vi "MAIN_launch_movie_acquisition.vi"(3 "error in":errorcluster, 4 "Data cluster":T3 {"Global parameters"."# repetitions" min=0; "Global parameters"."Dt (s)" min=0 step=1; "Global parameters"."Filter list" items=["ET665lp", "zet405/488/561/640m", "None", "None", "None", "None"]}, 5 "queue CAMERA":refnum<queue>) -> (1 "error out":errorcluster, 2 "Next task":T1)   [LabVIEW 2015]
uses:
  CONTROLS/Global parameters.ctl
  CONTROLS/Q_camera_element.ctl
  CONTROLS/Q_main_element.ctl
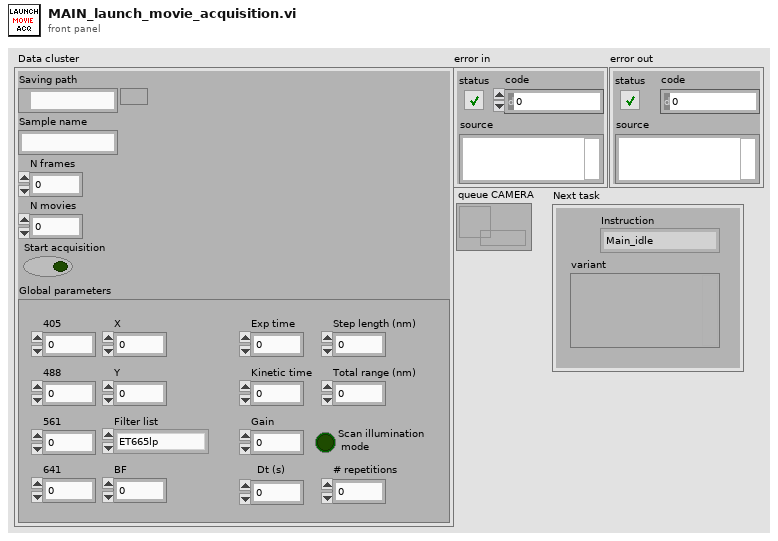
[diagram p1: front panel]
types:
  T1 = typedef "Q_main_element.ctl" = cluster{"variant":variant, "Instruction":enum16{"Main_idle", "Main_initialize", "Main_initialize_TDMS", "Main_initialize_Queue", "Main_error", "Main_DAQ_initialization_results", "Main_ASI_initialization_results", "Main_Piezo_initialization_results", "Main_Valve_initialization_results", "Main_Pump_initialization_results", "Main_CAMERA_initialization_results", "Main_FPGA_initialization_results", "Main_DAQ_error", "Main_ASI_error", "Main_Piezo_error", "Main_CAMERA_error", "Main_Valve_error", "Main_Pump_error", "Main_FPGA_error", "Main_start_acquiring", "Main_not_acquiring", "Main_acquiring", "Main_stop_acquiring", "Main_change_exposure", "Main_change_z_scan_parameters", "Main_define_ROI", "Main_define_mosaic", "Main_read_kinetic_time", "Main_cooler", "Main_read_temperature", "Main_save_XY", "Main_load_XY", "Main_discard_XY", "Main_move_to_XY", "Main_measure_QPD", "Main_autofocus_calibration", "Main_autofocus_initialization", "Main_autofocus_stop", "Main_save_PID", "Main_change_H_valve_position", "Main_two_way_valve", "Main_save_movie", "Main_init_single_scan", "Main_single_scan", "Main_stop_single_scan", "Main_merFISH_illumination_parameters", "Main_merFISH_buffer_probe_list", "Main_merFISH_injections_procedure", "Main_merFISH_save_setpoint", "Main_merFISH_DAPI_parameters", "Main_merFISH_Brightfield_parameters", "Main_merFISH_save_embryo_ROI", "Main_merFISH_init", "Main_merFISH_resume", "Main_merFISH_start_autofocus", "Main_merFISH_open_close_valve_merFISH", "Main_merFISH_open_close_valve_photobleaching", "Main_merFISH_hybridization", "Main_merFISH_move_to_ROI", "Main_merFISH_wait_stabilization", "Main_merFISH_move_to_REF", "Main_merFISH_scan", "Main_merFISH_photobleaching_injection", "Main_merFISH_photobleaching", "Main_merFISH_send_email", "Main_merFISH_close", "Main_STOP"}}
  T2 = typedef "Global parameters.ctl" = cluster{"405":dbl, "488":dbl, "561":dbl, "641":dbl, "BF":dbl, "X":dbl, "Y":dbl, "Filter list":u16, "Exp time":sgl, "Kinetic time":sgl, "Gain":i32, "Step length (nm)":u32, "Total range (nm)":u32, "Scan illumination\n mode":bool, "Dt (s)":i32, "# repetitions":i32}
  T3 = cluster{"Saving path":path, "Sample name":string, "N frames":i32, "N movies":i32, "Start acquisition":bool, "Global parameters":T2}
  T4 = typedef "Q_camera_element.ctl" = cluster{"variant":variant, "Instruction":enum16{"CAMERA_idle", "CAMERA_initialize", "CAMERA_error", "CAMERA_security_stop", "CAMERA_not_acquiring", "CAMERA_acquiring", "CAMERA_start_acquiring", "CAMERA_stop_acquiring", "CAMERA_change_exposure", "CAMERA_define_ROI", "CAMERA_cooler", "CAMERA_acquire_movie", "CAMERA_init_scan", "CAMERA_check_image_scan", "CAMERA_close_scan", "CAMERA_init_merFISH", "CAMERA_start_acquiring_merFISH", "CAMERA_close_scan_merFISH", "CAMERA_close_merFISH", "CAMERA_STOP"}}
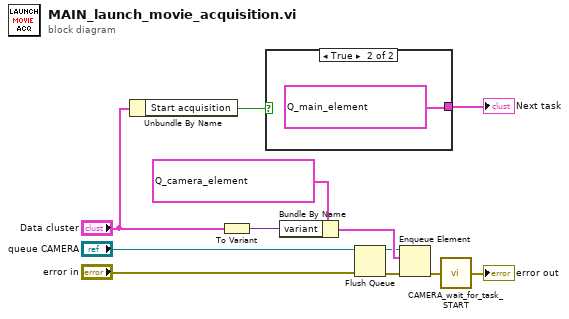
[diagram p0: block diagram]
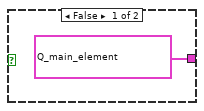
[diagram p2: hidden frame]
diagram:
  n1 = Unbundle By Name("Data cluster") -> ("Start acquisition"=w2:bool)
  n2 = To Variant(anything="Data cluster") -> (Variant=w8:variant)
  n3 = case shown="True" w2 {
    tunnel: [T1 {"variant"=variant, "Instruction"=enum."Main_not_acquiring"} ("Q_main_element") T1 {"variant"=variant, "Instruction"=enum."Main_start_acquiring"} ("Q_main_element")] -> w1
    frame False {
    }
    frame True {
    }
  }
  "Next task" <- w1
  n4 = Bundle By Name(cluster=T4 {"variant"=variant, "Instruction"=enum."CAMERA_acquire_movie"} ("Q_ANDOR_element"), "variant"=w8) -> (w11:T4)
  n5 = Flush Queue(queue="queue CAMERA", error in (no error)="error in") -> (queue out=w9:refnum<queue>, error out=w10:errorcluster)  [unwired: 1 out]
  n6 = Enqueue Element(queue=w9, element=w11, error in (no error)=w10) -> (error out=w12:errorcluster)  [unwired: 1 in, 2 out]
  n7 = call "CAMERA_wait_for_task_START.vi"("error in"=w12) -> ("error out"=→"error out":errorcluster)
